vi "HIS_to_DAT.vi"() -> ()   [LabVIEW 2015]
panel:
  in  "CERENKOV":bool
  in  "BRUIT":bool
  in  "BASE":bool
  in  "CERENKOV_path":path
  in  "BRUIT_path":path
  in  "stop_vi":bool
  in  "Selected images":dbl[](array[numeric])
  in  "ABS":bool
  in  "All":bool
  in  "select":bool caption="Lock"
  in  "Save":bool
  in  "BASE_path":path
  in  "ABS_path":path
  out "CERENKOV DAT":dbl[][](graph)
  in  "CERENKOVc":bool
  out "CERENKOV HIS":dbl[][](graph)
  out "BRUIT DAT":dbl[][](graph)
  in  "BRUITc":bool
  out "BRUIT HIS":dbl[][](graph)
  out "BASE DAT":dbl[][](graph)
  in  "BASEc":bool
  out "BASE HIS":dbl[][](graph)
  out "ABS DAT":dbl[][](graph)
  in  "ABSc":bool
  out "ABS HIS":dbl[][](graph)
  out "Slide":u8(slide) scale=0.0..100.0
  in  "Fast Forward":bool
  in  "Fast Reverse":bool
  in  "Stop":bool
  in  "Skip to End":bool
  in  "Skip to Beginning":bool
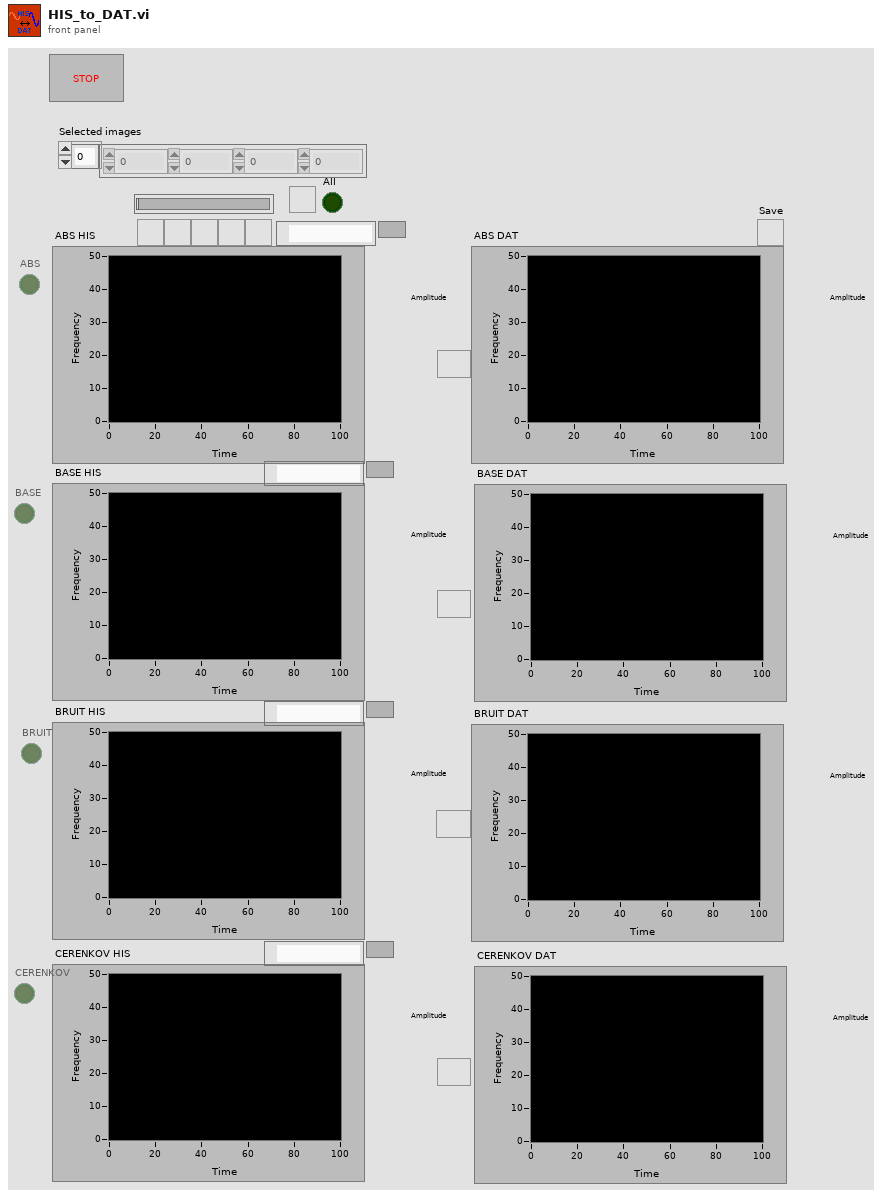
[diagram p1: front panel]
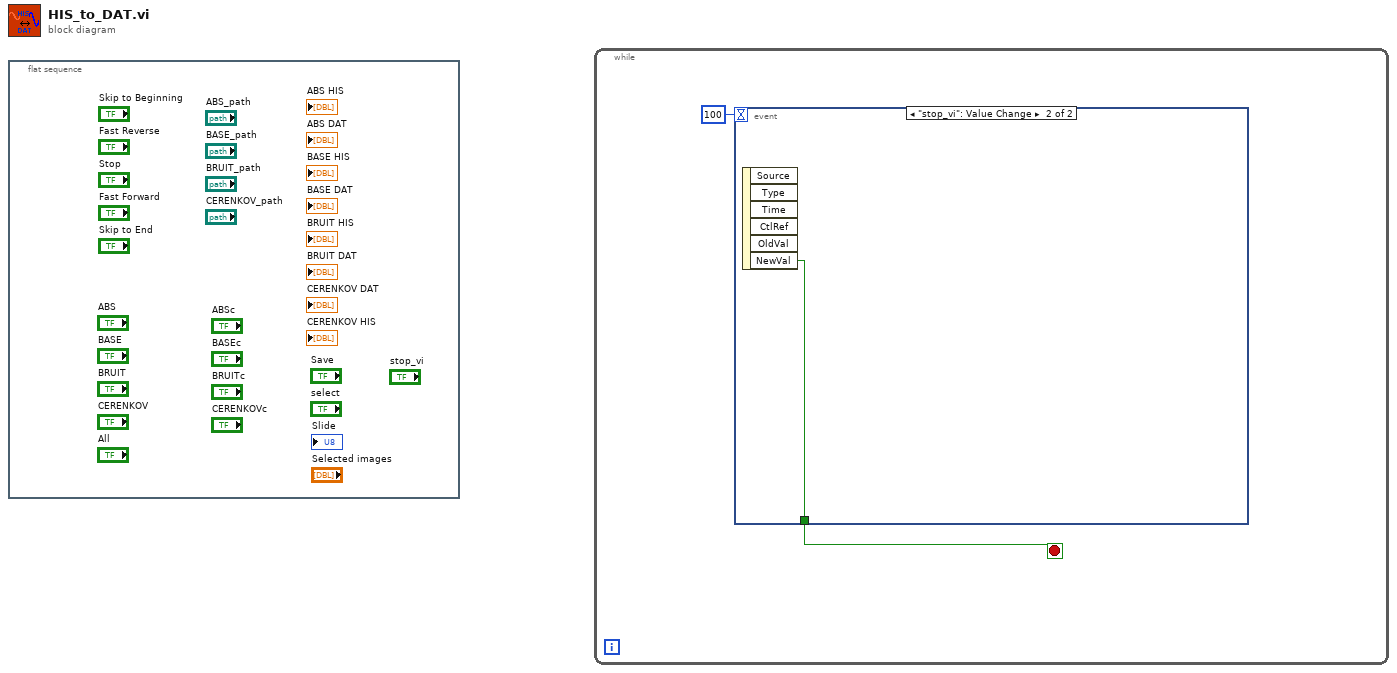
[diagram p0: block diagram]
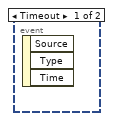
[diagram p2: hidden frame]
diagram:
  n1 = flat-sequence {
    frame #0 {
    }
  }
  n2 = while {
    stop <- w1 stop-if-true
    n3 = event shown="[1] \"stop_vi\": Value Change" {
      selector: _ -> [_ _]
      dyn-events: _ -> [_ _]
      timeout: 100 -> [_ _]
      tunnel: [_ w3] -> w1
      event Timeout {
        n4 = event-data() -> ()  [unwired: 1 in, 3 out]
      }
      event "stop_vi": Value Change {
        n5 = event-data() -> ("NewVal"=w3:bool)  [unwired: 1 in, 5 out]
      }
    }
  }
